vi "FdxGlobalDllPath.vi"() -> ()   [LabVIEW 2020, in "AIM664LV.lvlib"]
uses:
  AIM664LV.lvlib
panel:
  in  "FdxGlobalDllPath":path=path "aim_fdx.19.dll"
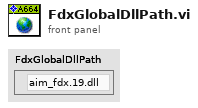
[diagram p1: front panel]
diagram:
